vi "OpenDevice.vi"(4 "RcvLen":u32, 5 "Enable2":bool=TRUE, 6 "DevIndex":u32, 7 "Enable1":bool=TRUE, 8 "error in (no error)":errorcluster caption="错误输入（无错误）", 9 "param":T2[](array[typedef]) {"ACR0" format="%x"}, 10 "Channels":u32[](array[numeric]), 11 "type":u16(ring)=2 items=["USB-CAN"=2, "USB-CAN2.0"=3]) -> (0 "error out":errorcluster caption="错误输出", 1 "bridge type":T1(ring) caption="中继类型：", 2 "Error info":string, 3 "open":bool)   [LabVIEW 2011]
uses:
  VIs/Param.ctl
  data/ControlCAN.dll
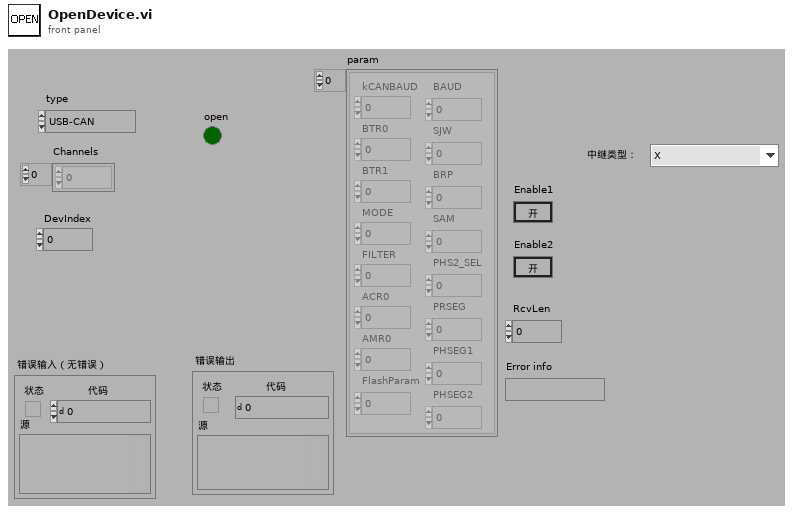
[diagram p1: front panel]
types:
  T1 = enum16{"X", "CAN1--->CAN2", "CAN1<----CAN2", "CAN1<---->CAN2"}
  T2 = typedef "Param.ctl" = cluster{"kCANBAUD":u8, "BTR0":u8, "BTR1":u8, "MODE":u8, "FILTER":u8, "ACR0":u32, "AMR0":u32, "FlashParam":u32, "BAUD":u32, "SJW":u8, "BRP":u8, "SAM":u8, "PHS2_SEL":u8, "PRSEG":u8, "PHSEG1":u8, "PHSEG2":u8}
  T3 = cluster{"AccCode":u32, "AccMask":u32, "Reserved":u32, "Filter":u8, "Timing0":u8, "Timing1":u8, "Mode":u8}
  T4 = enum32{"Bad", "Idle", "Run top level", "Running"}
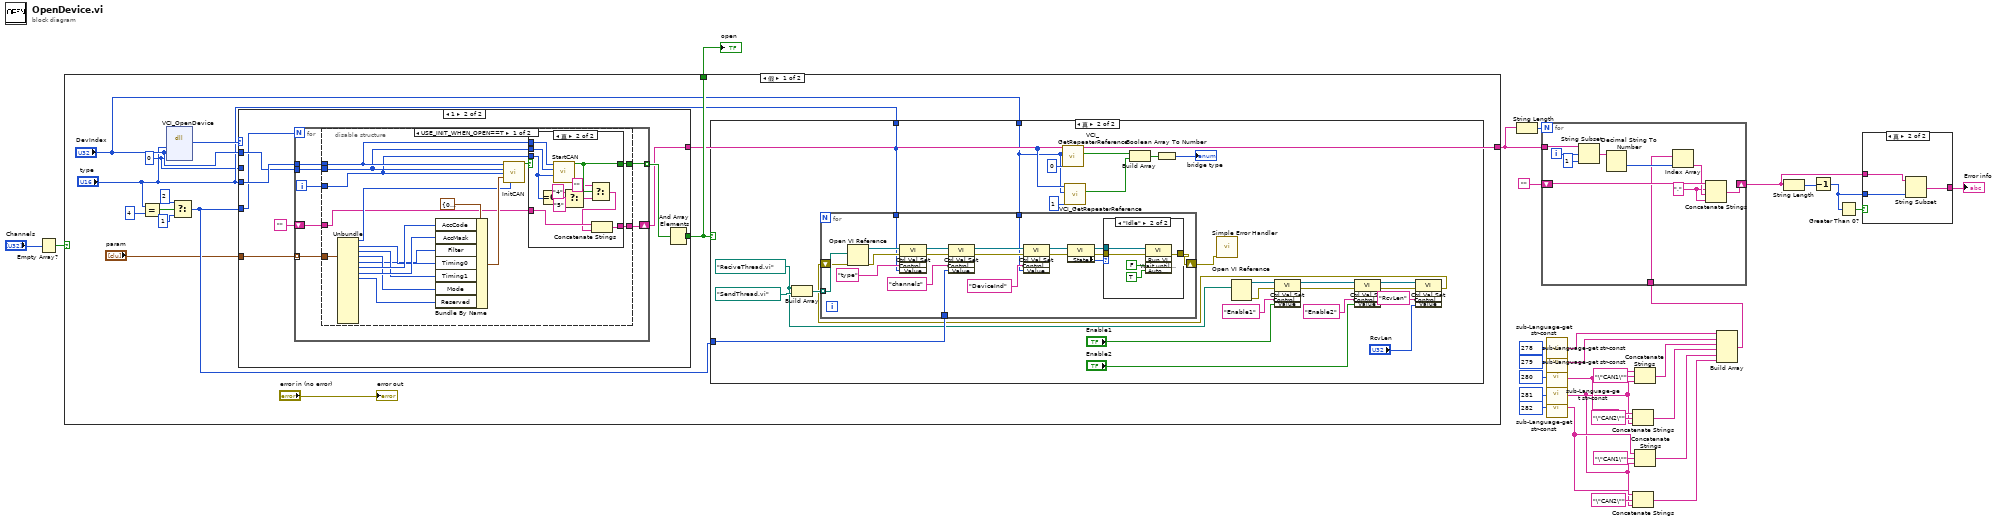
[diagram p0: block diagram]
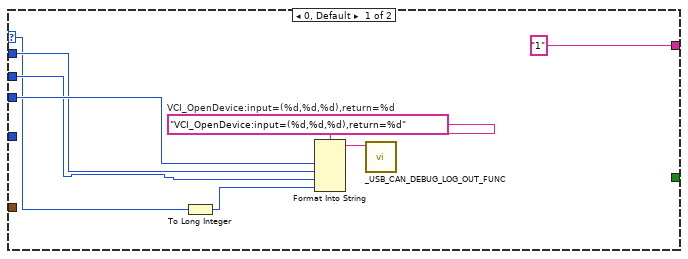
[diagram p5: hidden frame]
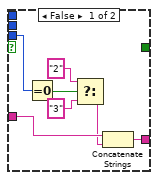
[diagram p6: hidden frame]
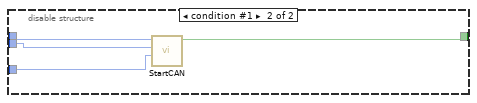
[diagram p7: hidden frame]
diagram:
  n1 = Empty Array?(array="Channels") -> (empty?=w28:bool)
  n2 = case shown="假" w28 {
    tunnel: [w41 _] -> w30
    tunnel: [w32 _] -> w26
    frame False {
      w31 = u32 0 ("DevIndex")
      n3 = Equal?(x="type", y=u16 4) -> (x = y?=w37:bool)
      n4 = dll-call lib="PTH1Qabs CUsers\nAdministratorDesktopV2.12(等同2.04）dataControlCAN.dll" fn="VCI_OpenDevice"("DevType"="type", "DevIndex"="DevIndex", "Reserved"=w31) -> ("返回类型"=w43:u32)  [unwired: 6 in, 2 out]
      n5 = Select(t=2 ("y"), s=w37, f=1 ("y")) -> (s? t:f=w34:i32)
      n6 = case shown="1" w43 {
        selector: w43 -> [w97 _]
        tunnel: "type" -> [w100 w110]
        tunnel: [_ w111] -> w41
        tunnel: "DevIndex" -> [w99 w109]
        tunnel: w34 -> [_ w107]
        tunnel: "param" -> [_ w106]
        tunnel: ["1" w104] -> w32
        tunnel: w31 -> [w98 _]
        frame 0, Default {
          w101 = "VCI_OpenDevice:input=(%d,%d,%d),return=%d"  # VCI_OpenDevice:input=(%d,%d,%d),return=%d
          n7 = To Long Integer(number=w97) -> (32bit integer=w96:i32)
          n8 = Format Into String(format string=w101, w100, w99, w98, w96) -> (resulting string=w102:string)  [unwired: 2 in, 1 out]
          n9 = call "_USB_CAN_DEBUG_LOG_OUT_FUNC.vi"("Info"=w102) -> ()  [unwired: 11 in]
        }
        frame 1 {
          n10 = for {
            N: w107 -> [_]
            tunnel: w110 -> [w116]
            tunnel: w109 -> [w115]
            tunnel: [w118] -> w108 mode=indexing
            tunnel: w106 -> [w117] mode=indexing
            shift-right: [w112] -> w104
            shift-left: "" -> [w113]
            i -> [w114]
            n11 = disable-structure shown="USE_INIT_WHEN_OPEN==T" {
              disable-tunnel: [w136 w156] -> w118
              disable-tunnel: w117 -> [w135 _]
              disable-tunnel: w116 -> [w127 w159]
              disable-tunnel: w115 -> [w126 w158]
              disable-tunnel: w114 -> [w125 w157]
              disable-tunnel: w113 -> [w120 _]
              disable-tunnel: [w119 _] -> w112
              frame condition #0 (active) {
                n12 = Unbundle(w135) -> ("kCANBAUD"=w121:u8, "BTR0"=w132:u8, "BTR1"=w131:u8, "MODE"=w130:u8, "FILTER"=w123:u8, "ACR0"=w134:u32, "AMR0"=w133:u32, "FlashParam"=w124:u32)  [unwired: 8 out]
                n13 = Bundle By Name(cluster=T3 {"AccCode"=0, "AccMask"=0, "Reserved"=0, "Filter"=0, "Timing0"=0, "Timing1"=0, "Mode"=0} ("pInitConfig"), "AccCode"=w134, "AccMask"=w133, "Filter"=w123, "Timing0"=w132, "Timing1"=w131, "Mode"=w130, "Reserved"=w124) -> (w129:T3)
                n14 = call "InitCAN.vi"("DeviceType"=w127, "DeviceInd"=w126, "CANInd"=w125, "pInitConfig"=w129, "br"=w121) -> ("Success"=w128:bool)  [unwired: 9 in, 1 out]
                n15 = case shown="真" w128 {
                  tunnel: [_ w149] -> w136
                  tunnel: w127 -> [_ w155]
                  tunnel: w126 -> [_ w154]
                  tunnel: w125 -> [w143 w150]
                  tunnel: w120 -> [w139 w146]
                  tunnel: [w137 w144] -> w119
                  frame False {
                    n16 = Equal To 0?(x=w143) -> (x = 0?=w142:bool)
                    n17 = Select(t="2", s=w142, f="3") -> (s? t:f=w138:string)
                    n18 = Concatenate Strings(w139, w138) -> (w137:string)
                  }
                  frame True {
                    n19 = Equal To 0?(x=w150) -> (x = 0?=w153:bool)
                    n20 = call "StartCAN.vi"("CANInd"=w150, "DeciceInd"=w154, "DeviceType"=w155) -> ("Valid"=w149:bool)  [unwired: 7 in, 1 out]
                    n21 = Select(t="4", s=w153, f="5") -> (s? t:f=w147:string)
                    n22 = Select(t="", s=w149, f=w147) -> (s? t:f=w145:string)
                    n23 = Concatenate Strings(w146, w145) -> (w144:string)
                  }
                }
              }
              frame condition #1 {
                n24 = call "StartCAN.vi"("CANInd"=w157, "DeciceInd"=w158, "DeviceType"=w159) -> ("Valid"=w156:bool)  [unwired: 7 in, 1 out]
              }
            }
          }
          n25 = And Array Elements(Boolean array=w108) -> (logical AND=w111:bool)
        }
      }
      n26 = case shown="真" w41 {
        tunnel: "type" -> [_ w49]
        tunnel: "DevIndex" -> [_ w44]
        tunnel: w34 -> [_ w67]
        frame False {
        }
        frame True {
          w66 = path "ReciveThread.vi" ("VI路径")
          n27 = Build Array(w66, path "SendThread.vi" ("VI路径")) -> (w69:path[])
          n28 = call "VCI_GetRepeaterReference.vi"("CANIndex"=u32 0, "DevIndex"=w44, "DevType"=w49) -> ("On"=w45:bool)  [unwired: 6 in, 2 out]
          n29 = call "VCI_GetRepeaterReference.vi"("CANIndex"=u32 1, "DevIndex"=w44, "DevType"=w49) -> ("On"=w46:bool)  [unwired: 6 in, 2 out]
          n30 = Build Array(w45, w46) -> (w48:bool[])
          n31 = Boolean Array To Number(Boolean array=w48) -> (number=→"bridge type":u32)
          n32 = Open VI Reference(vi path=w66) -> (vi reference=w65:refnum<vi>, error out=w64:errorcluster)  [unwired: 5 in]
          n33 = invoke class="VI" method="Ctrl Val.Set"(reference=w65, error in=w64, "Control Name"="Enable1" ("控件名"), "Value"="Enable1") -> (reference out=w60:refnum<vi>, error out=w59:errorcluster)  [unwired: 1 in, 3 out]
          n34 = invoke class="VI" method="Ctrl Val.Set"(reference=w60, error in=w59, "Control Name"="Enable2" ("控件名"), "Value"="Enable2") -> (reference out=w56:refnum<vi>, error out=w55:errorcluster)  [unwired: 1 in, 3 out]
          n35 = invoke class="VI" method="Ctrl Val.Set"(reference=w56, error in=w55, "Control Name"="RcvLen" ("控件名"), "Value"="RcvLen") -> (error out=w52:errorcluster)  [unwired: 1 in, 4 out]
          n36 = for {
            tunnel: w69 -> [w83] mode=indexing
            tunnel: w49 -> [w79]
            tunnel: w44 -> [w73]
            tunnel: w67 -> [w72]
            shift-right: [w71] -> w57
            shift-left: w52 -> [w70]
            n37 = Open VI Reference(vi path=w83, error in (no error)=w70) -> (vi reference=w89:refnum<vi>, error out=w88:errorcluster)  [unwired: 4 in]
            n38 = invoke class="VI" method="Ctrl Val.Set"(reference=w89, error in=w88, "Control Name"="type" ("控件名"), "Value"=w79) -> (reference out=w86:refnum<vi>, error out=w85:errorcluster)  [unwired: 1 in, 3 out]
            n39 = invoke class="VI" method="Ctrl Val.Set"(reference=w86, error in=w85, "Control Name"="channels" ("控件名"), "Value"=w72) -> (reference out=w76:refnum<vi>, error out=w75:errorcluster)  [unwired: 1 in, 3 out]
            n40 = invoke class="VI" method="Ctrl Val.Set"(reference=w76, error in=w75, "Control Name"="DeviceInd" ("控件名"), "Value"=w73) -> (reference out=w78:refnum<vi>, error out=w77:errorcluster)  [unwired: 1 in, 3 out]
            n41 = property class="VI"(reference=w78, error in=w77) -> (reference out=w81:refnum<vi>, error out=w80:errorcluster, "Exec.State"=w82:T4)
            n42 = case shown="\"Idle\"" w82 {
              tunnel: w81 -> [_ w93]
              tunnel: w80 -> [w90 w92]
              tunnel: [w90 w91] -> w71
              frame "Bad", Default {
              }
              frame "Idle" {
                n43 = invoke class="VI" method="Run VI"(reference=w93, error in=w92, "Wait until done"=FALSE ("结束前等待"), "Auto Dispose Ref"=TRUE ("自动销毁引用")) -> (error out=w91:errorcluster)  [unwired: 1 in, 4 out]
              }
            }
          }
          n44 = call <vilib>:"Simple Error Handler.vi"("error in (no error)"=w57) -> ()  [unwired: 4 in, 5 out]
        }
      }
      "error out" <- "error in (no error)"
    }
    frame True {
    }
  }
  "open" <- w30
  n45 = String Length(string=w26) -> (length=w27:i32)
  n46 = call "sub-Language-get str-const.vi"("sid"=u32 278) -> ("str"=w14:string)
  n47 = call "sub-Language-get str-const.vi"("sid"=u32 279) -> ("str"=w13:string)
  n48 = call "sub-Language-get str-const.vi"("sid"=u32 280) -> ("str"=w9:string)
  n49 = call "sub-Language-get str-const.vi"("sid"=u32 281) -> ("str"=w4:string)
  n50 = call "sub-Language-get str-const.vi"("sid"=u32 282) -> ("str"=w5:string)
  n51 = Concatenate Strings(w9, "\"CAN2\"" ("字符串"), w4) -> (w8:string)
  n52 = Concatenate Strings(w5, "\"CAN2\"" ("字符串"), w4) -> (w2:string)
  n53 = Concatenate Strings(w9, "\"CAN1\"" ("字符串"), w4) -> (w10:string)
  n54 = Concatenate Strings(w5, "\"CAN1\"" ("字符串"), w4) -> (w3:string)
  n55 = Build Array(w14, w13, w10, w8, w3, w2) -> (w1:string[])
  n56 = for {
    N: w27 -> [_]
    tunnel: w26 -> [w169]
    shift-right: [w162] -> w22
    shift-left: "" -> [w164]
    tunnel: w1 -> [w161]
    i -> [w168]
    w160 = "," ("字符串")
    n57 = String Subset(string=w169, offset (0)=w168, length (rest)=1 ("长度（剩余）")) -> (substring=w166:string)
    n58 = Decimal String To Number(string=w166) -> (number=w165:i32)  [unwired: 2 in, 1 out]
    n59 = Index Array(array=w161, index=w165) -> (element=w163:string)
    n60 = Concatenate Strings(w164, w160, w163, w160) -> (w162:string)
  }
  n61 = String Length(string=w22) -> (length=w24:i32)
  n62 = Decrement(x=w24) -> (x-1=w21:i32)
  n63 = Greater Than 0?(x=w21) -> (x > 0?=w23:bool)
  n64 = case shown="真" w23 {
    tunnel: w22 -> [_ w172]
    tunnel: w21 -> [_ w171]
    tunnel: [_ w170] -> w20
    frame False {
    }
    frame True {
      n65 = String Subset(string=w172, length (rest)=w171) -> (substring=w170:string)  [unwired: 1 in]
    }
  }
  "Error info" <- w20
